vi "XIPIN_Chroma_Resampler_4_0.vi"   [LabVIEW 2017]
doc: "The Xilinx Chroma Resampler LogiCORE provides users with an easy-to-use IP block for converting between chroma subsampling formats of 4:4:4, 4:2:2, and 4:2:0.\n------------------------------------\n<b>Need License</b> : Yes\n<b>Interface</b> : AXI4 AXI4-Stream"
uses:
  <vilib>/rvi/XilinxIP/XIPIN_XNode/niFpgaXIPIN.xnode
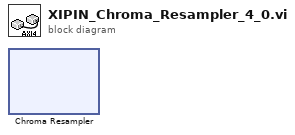
[diagram p0: block diagram]
diagram:
  n1 = xnode ("Chroma Resampler")() -> ()
